vi "OUTPUT.vi"(8 "error in (no error)":errorcluster) -> (0 "error out":errorcluster, 3 "COM":string)   [LabVIEW 2020, in "GPP.lvlib"]
uses:
  GPP.lvlib
  <vilib>/Utility/config.llb/Read Key (String).vi
  <vilib>/Utility/config.llb/NI_LVConfig.lvlib
panel:
  in  "ON/OFF":bool
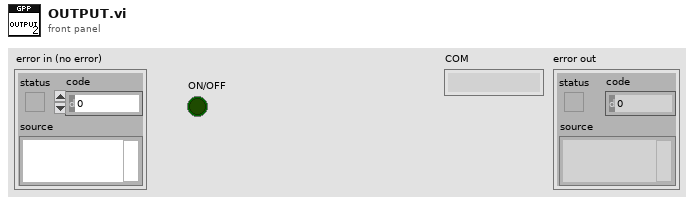
[diagram p1: front panel]
types:
  T1 = typedef "NI_LVConfig.lvlib/Config Data RefNum.ctl" = refnum<k1>
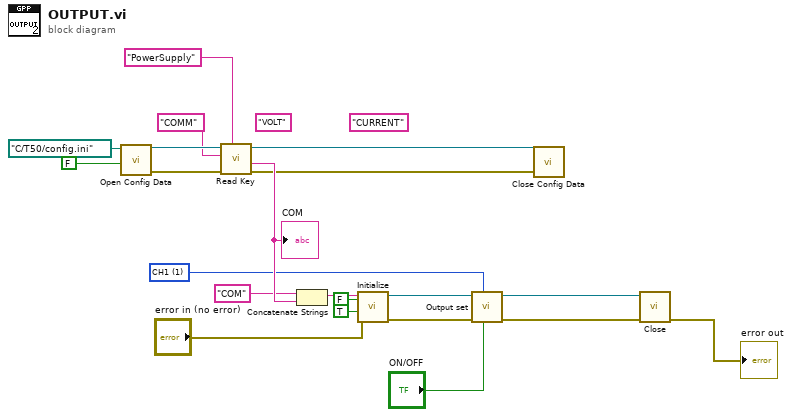
[diagram p0: block diagram]
diagram:
  w4 = u16 1 items=["CH1"=1, "CH2"=2, "CH3"=3, "CH4"=4] ("Channel  (1: CH1)")
  (unwired) "CURRENT" ("key")
  (unwired) "VOLT" ("key")
  n1 = call <vilib>:"Open Config Data.vi"("create file if necessary (T)"=FALSE, "configuration file path"=path "C:/T50/config.ini") -> ("error out"=w20:errorcluster, "refnum"=w19:T1)  [unwired: 7 in, 1 out]
  n2 = call-poly <vilib>:"Read Key.vi"("section"="PowerSupply", "error in (no error)"=w20, "key"="COMM", "refnum"=w19) -> ("error out"=w8:errorcluster, "value"=w16:string, "refnum out"=w7:T1)  [unwired: 4 in, 1 out]
  "COM" <- w16
  n3 = Concatenate Strings("COM" ("string"), w16) -> (w13:string)
  n4 = call "Initialize.vi"("error in (no error)"="error in (no error)", "Reset (True)"=TRUE, "ID Query (True)"=FALSE, "VISA resource name"=w13) -> ("error out"=w6:errorcluster, "VISA resource name out"=w5:refnum<visa-resource-name>)  [unwired: 5 in, 1 out]
  n5 = call "Output set.vi"("Output(T:ON F:OFF)"="ON/OFF", "Channel  (1: CH1)"=w4, "error in (no error)"=w6, "VISA resource in"=w5) -> ("error out"=w2:errorcluster, "VISA resource name out"=w3:refnum<visa-resource-name>)  [unwired: 6 in]
  n6 = call <vilib>:"Close Config Data.vi"("error in (no error)"=w8, "refnum"=w7) -> ()  [unwired: 8 in, 2 out]
  n7 = call "Close.vi"("error in (no error)"=w2, "VISA resource name"=w3) -> ("error out"=→"error out":errorcluster)  [unwired: 9 in]
